vi "Array-Last Element.vi"(1 "V":dbl[](array[numeric])) -> (0 "Numeric":i32)   [LabVIEW 2015]
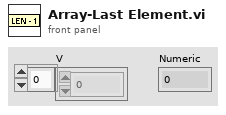
[diagram p1: front panel]
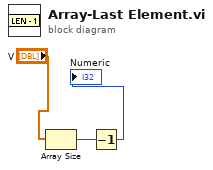
[diagram p0: block diagram]
diagram:
  n1 = Array Size(array="V") -> (size(s)=w1:i32)
  n2 = Decrement(x=w1) -> (x-1=→"Numeric":i32)
